vi "PAM Get Time Stamp.vi"(1 "icListen Metadata":T1 {"Temperature" format="%#_3g"; "Humidity" format="%_3f"}) -> (0 "Time Stamp":timestamp)   [LabVIEW 2020]
doc: "This VI convert a date/time string back to a time stamp."
uses:
  <vilib>/Utility/miscctls.llb/LVDateTimeRec.ctl
panel:
  in  "Error In":errorcluster
  out "Error Out":errorcluster
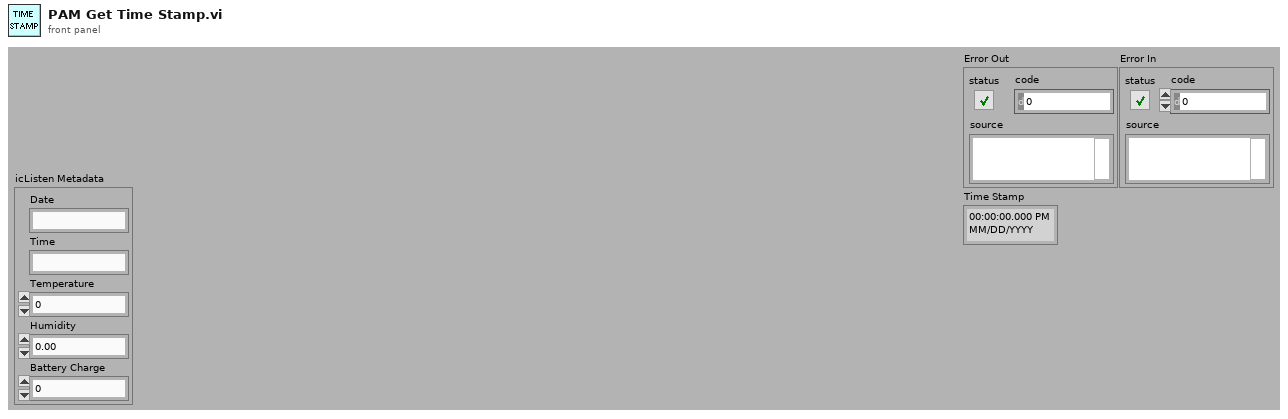
[diagram p1: front panel]
types:
  T1 = cluster{"Date":string, "Time":string, "Temperature":dbl, "Humidity":dbl, "Battery Charge":i32}
  T2 = typedef "LVDateTimeRec.ctl" = cluster{"fractional second":dbl, "second":i32, "minute":i32, "hour":i32, "day of month":i32, "month":i32, "year":i32, "day of week":i32, "day of year":i32, "DST":i32}
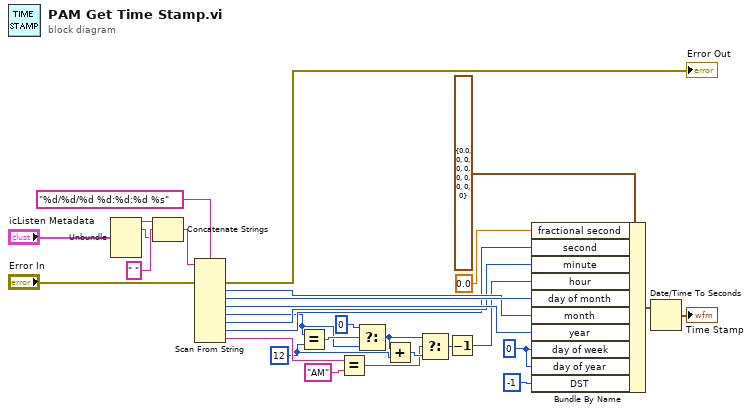
[diagram p0: block diagram]
diagram:
  w19 = 12 ("y")
  w7 = 0
  n1 = Unbundle("icListen Metadata") -> ("Date"=w12:string, "Time"=w11:string)  [unwired: 3 out]
  n2 = Concatenate Strings(w12, " " ("string"), w11) -> (w14:string)
  n3 = Scan From String "Scan From String"(format string="%d/%d/%d %d:%d:%d %s", input string=w14, error in="Error In") -> (error out=→"Error Out":errorcluster, output 1=w27:i32, output 2=w28:i32, output 3=w26:i32, output 4=w17:i32, output 5=w25:i32, output 6=w24:i32, output 7=w23:string)  [unwired: 8 in, 2 out]
  n4 = Equal?(x=w17, y=w19) -> (x = y?=w18:bool)
  n5 = Equal?(x=w23, y="AM") -> (x = y?=w20:bool)
  n6 = Select(t=0, s=w18, f=w17) -> (s? t:f=w16:i32)
  n7 = Add(x=w16, y=w19) -> (x+y=w21:i32)
  n8 = Select(t=w16, s=w20, f=w21) -> (s? t:f=w3:i32)
  n9 = Decrement(x=w3) -> (x-1=w2:i32)
  n10 = Bundle By Name(cluster=T2 {"fractional second"=0.0, "second"=0, "minute"=0, "hour"=0, "day of month"=0, "month"=0, "year"=0, "day of week"=0, "day of year"=0, "DST"=0} ("date time rec"), "fractional second"=0.0, "second"=w24, "minute"=w25, "hour"=w2, "day of month"=w28, "month"=w27, "year"=w26, "day of week"=w7, "day of year"=w7, "DST"=-1) -> (w8:T2)
  n11 = Date/Time To Seconds(2:w8) -> (0:→"Time Stamp":timestamp)  [unwired: 1 in]
